vi "Scan_junk.vi"(0 "DMM ref":refnum<visa-resource-name>, 1 "output cluster":cluster{"Timeout":i32, "Channel number":i32}, 2 "P_current_count":i32, 3 "N_current_count":i32, 5 "DMM error":errorcluster, 7 "Current Sense \nResitance Array":dbl[](array[numeric])=[1.0032214, 1.00250644, 1.00234822, 1.0040944, 1.0017711, 1.00229431, 1.00344206, 1.00482066, 1.00381056, 1.00290978, 1.00333016, 1.00367587], 9 "ESP32 ref":refnum<visa-resource-name>, 11 "ESP32 error":errorcluster, 12 "current_mode":u8[](array[numeric])=[0, 0, 0, 0, 0, 0, 0, 0, 0, 0, 0]) -> (4 "DMM ref":refnum<visa-resource-name>, 6 "DMM error":errorcluster, 8 "Measurements":dbl[](array[numeric]), 10 "ESP32 ref":refnum<visa-resource-name>, 13 "Timout?":bool, 14 "Time out count":i32, 15 "Measurements 2":dbl[](array[numeric]))   [LabVIEW 2023]
uses:
  <instrlib>/Agilent 3446X Series/Agilent 3446X Series.lvlib
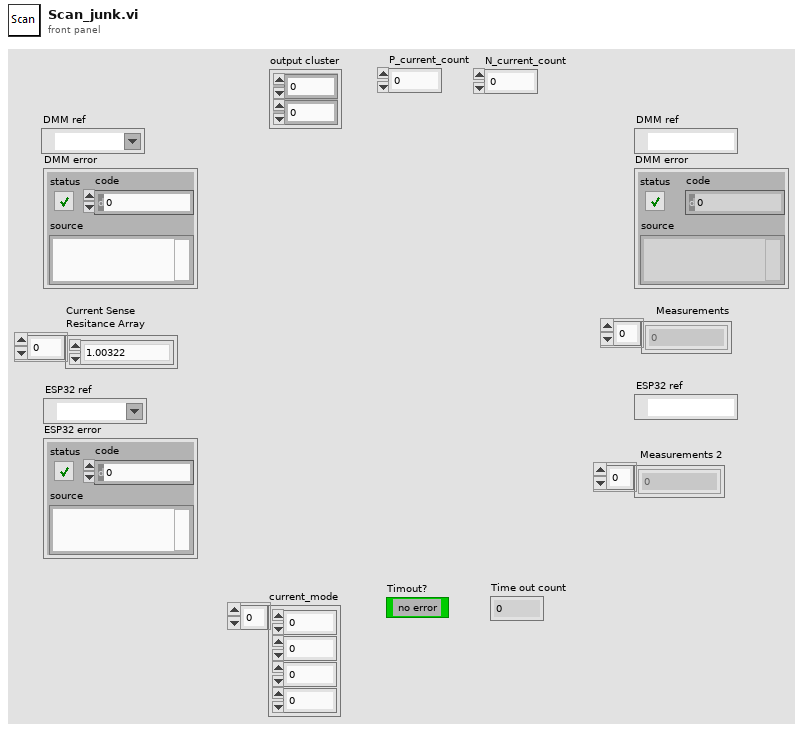
[diagram p1: front panel]
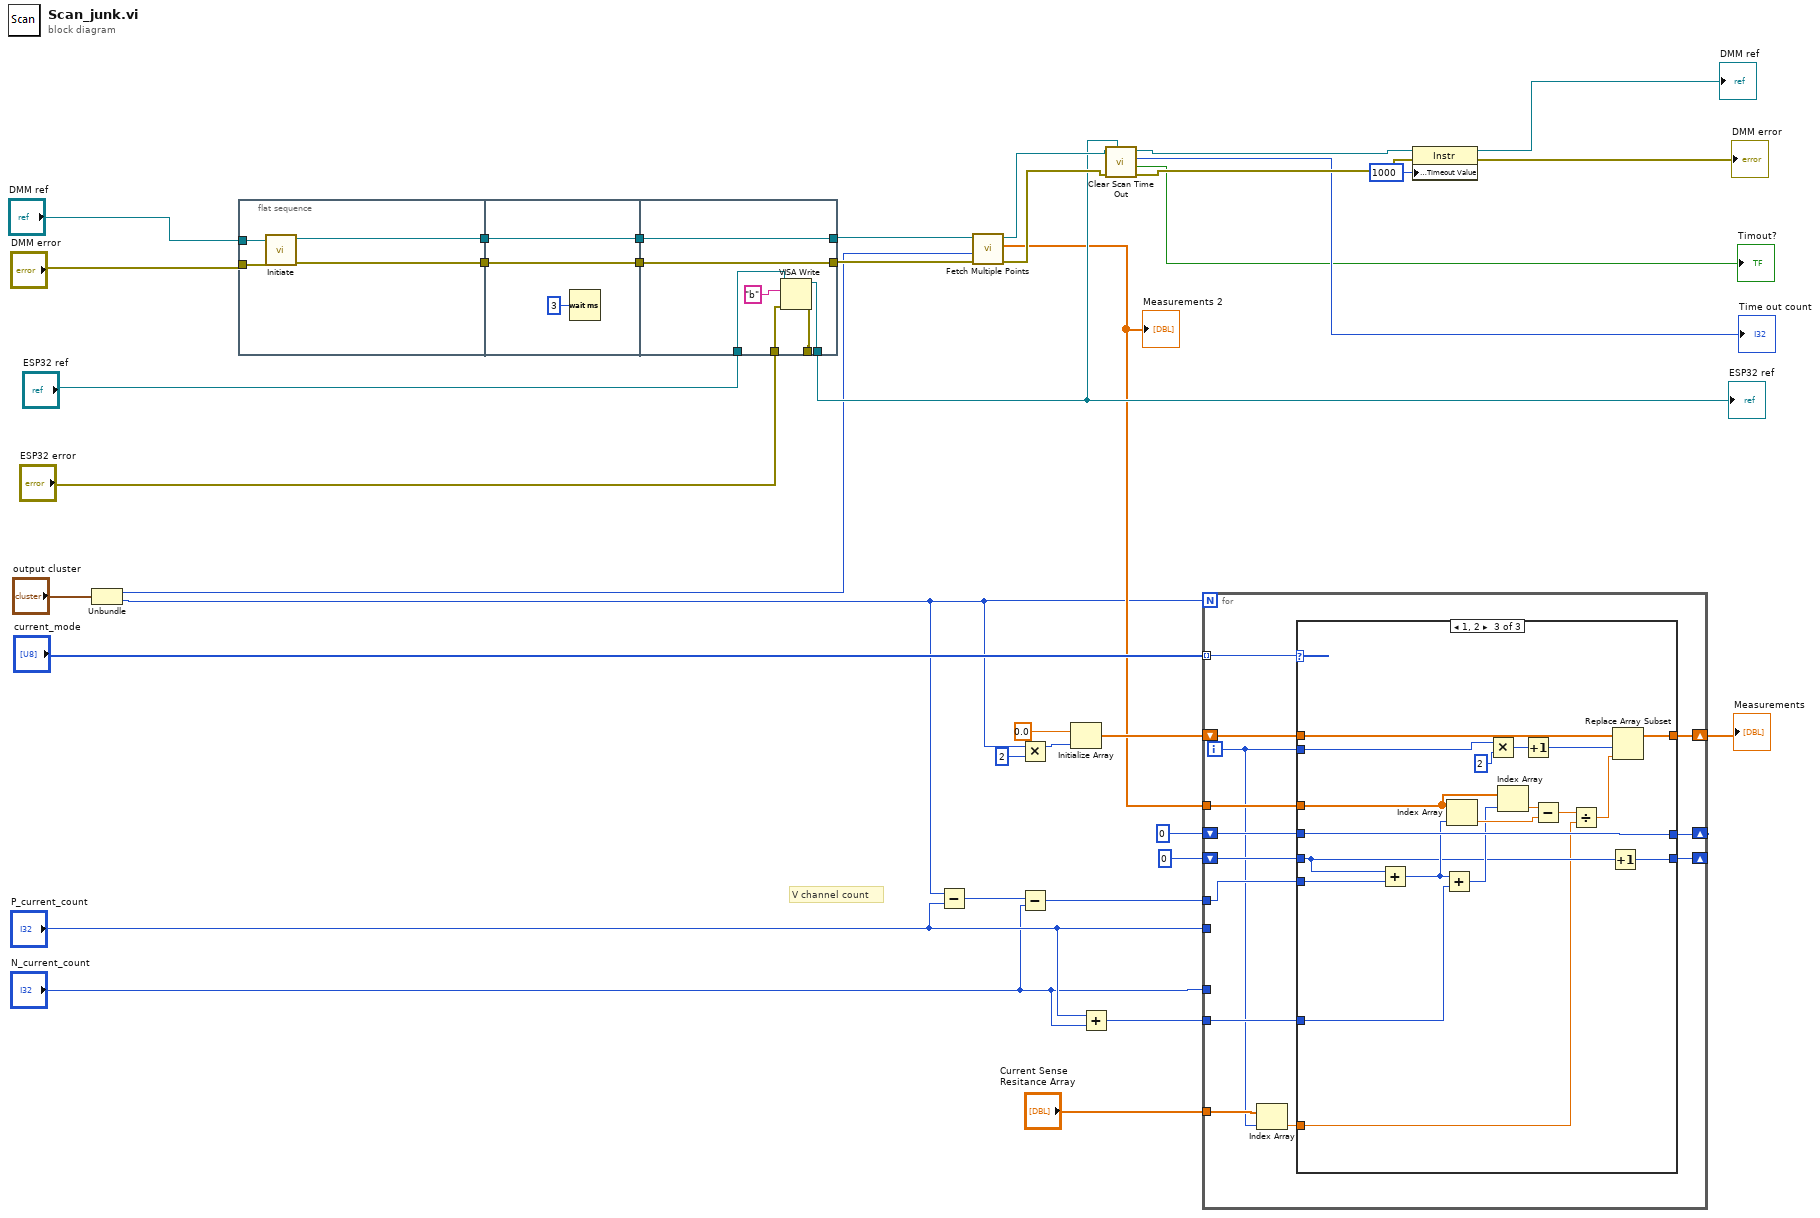
[diagram p0: block diagram]
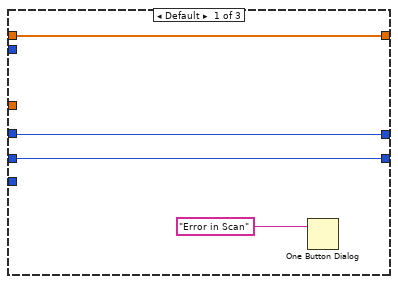
[diagram p2: hidden frame]
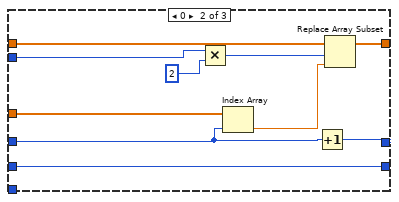
[diagram p3: hidden frame]
diagram:
  # "V channel count"
  n1 = Unbundle("output cluster") -> ("Timeout"=w1:i32, "Channel number"=w2:i32)
  n2 = flat-sequence {
    tunnel: [w42] -> w38
    tunnel: [w41] -> w37
    tunnel: "DMM ref" -> [w40]
    tunnel: "DMM error" -> [w39]
    tunnel: w38 -> [w45]
    tunnel: [w45] -> w36
    tunnel: w37 -> [w44]
    tunnel: [w44] -> w35
    tunnel: w36 -> [w52]
    tunnel: w35 -> [w51]
    tunnel: "ESP32 ref" -> [w50]
    tunnel: "ESP32 error" -> [w49]
    tunnel: [w48] -> w21
    tunnel: [w47] -> _
    tunnel: [w52] -> w34
    tunnel: [w51] -> w33
    frame #0 {
      n3 = call <instrlib>:"Initiate.vi"("error in (no error)"=w39, "VISA resource name"=w40) -> ("error out"=w42:errorcluster, "VISA resource name out"=w41:refnum<visa-resource-name>)  [unwired: 8 in]
    }
    frame #1 {
      n4 = Wait (ms)(milliseconds to wait=u32 3) -> ()  [unwired: 1 out]
    }
    frame #2 {
      n5 = VISA Write(VISA resource name=w50, write buffer="b" ("data in"), error in (no error)=w49) -> (VISA resource name out=w48:refnum<visa-resource-name>, error out=w47:errorcluster)  [unwired: 1 out]
    }
  }
  n6 = Subtract(x=w2, y="P_current_count") -> (x-y=w12:i32)
  n7 = call <instrlib>:"Fetch Multiple Points.vi"("error in (no error)"=w34, "Timeout (10000 ms)"=w1, "VISA resource name"=w33) -> ("error out"=w29:errorcluster, "Measurements"=w13:dbl[], "VISA resource name out"=w30:refnum<visa-resource-name>)  [unwired: 1 in, 5 out]
  "Measurements 2" <- w13
  n8 = Multiply(x=w2, y=2) -> (x*y=w17:i32)
  n9 = Subtract(x=w12, y="N_current_count") -> (x-y=w11:i32)
  n10 = Initialize Array(0.0 ("Measurement"), w17) -> (w15:dbl[])
  n11 = Add(x="P_current_count", y="N_current_count") -> (x+y=w6:i32)
  n12 = call "Clear Scan Time Out.vi"("ESP32 ref"=w21, "error in (no error)"=w29, "VISA Refnum in"=w30) -> ("error out"=w27:errorcluster, "error?"=→"Timout?":bool, "Time out count"=→"Time out count":i32, "VISA Refnum out"=w28:refnum<visa-resource-name>)  [unwired: 4 in, 1 out]
  n13 = for {
    N: w2 -> [_]
    shift-right: [w60] -> w5
    shift-left: w15 -> [w61]
    tunnel: "current_mode" -> [w65] mode=indexing
    tunnel: w13 -> [w64]
    tunnel: "P_current_count" -> [_]
    tunnel: "N_current_count" -> [_]
    tunnel: w11 -> [w57]
    shift-right: [w62] -> _
    shift-left: 0 ("index") -> [w63]
    shift-right: [w58] -> _
    shift-left: 0 ("index") -> [w59]
    tunnel: w6 -> [w56]
    tunnel: "Current Sense \nResitance Array" -> [w55]
    i -> [w54]
    n14 = Index Array(array=w55, index=w54) -> (element=w53:dbl)
    n15 = case shown="1, 2" w65 {
      tunnel: w64 -> [_ w79 w91]
      tunnel: w63 -> [w69 w77 w92]
      tunnel: [w69 w76 w92] -> w62
      tunnel: w54 -> [_ w74 w97]
      tunnel: w61 -> [w68 w75 w98]
      tunnel: [w68 w72 w94] -> w60
      tunnel: w59 -> [w67 w71 w84]
      tunnel: [w67 w71 w83] -> w58
      tunnel: w57 -> [_ _ w88]
      tunnel: w56 -> [_ _ w87]
      tunnel: w53 -> [_ _ w81]
      frame Default {
        n16 = One Button Dialog(message="Error in Scan") -> ()  [unwired: 1 in, 1 out]
      }
      frame 0 {
        n17 = Multiply(x=w74, y=2 ("x")) -> (x*y=w70:i32)
        n18 = Index Array(array=w79, index=w77) -> (element=w78:dbl)
        n19 = Increment(x=w77) -> (x+1=w76:i32)
        n20 = Replace Array Subset(array=w75, new element=w78, index=w70) -> (w72:dbl[])
      }
      frame 1, 2 {
        n21 = Add(x=w84, y=w88) -> (x+y=w86:i32)
        n22 = Add(x=w86, y=w87) -> (x+y=w85:i32)
        n23 = Index Array(array=w91, index=w86) -> (element=w89:dbl)
        n24 = Multiply(x=w97, y=2 ("x")) -> (x*y=w95:i32)
        n25 = Index Array(array=w91, index=w85) -> (element=w90:dbl)
        n26 = Increment(x=w95) -> (x+1=w93:i32)
        n27 = Subtract(x=w90, y=w89) -> (x-y=w82:dbl)
        n28 = Divide(x=w82, y=w81) -> (x/y=w80:dbl)
        n29 = Increment(x=w84) -> (x+1=w83:i32)
        n30 = Replace Array Subset(array=w98, new element=w80, index=w93) -> (w94:dbl[])
      }
    }
  }
  "Measurements" <- w5
  n31 = property class="Instr"(reference=w28, error in=w27, "General Settings:Timeout Value"=u32 1000) -> (reference out=→"DMM ref":refnum<visa-resource-name>, error out=→"DMM error":errorcluster)
  "ESP32 ref" <- w21
